vi "_test LoadUnload.vi"() -> ()   [LabVIEW 2020]
uses:
  C:/Users/Administrator/Desktop/GIT/Ballard-Arinc-429-XML-Generator/Source/Assemblies/Ballard_Parameter_ni/bin/Debug/Parameters_Arinc429_XML_Tools.dll
  Source/Assemblies/Ballard_Parameter_ni/bin/Debug/Parameters_Arinc429_XML_Tools.dll
panel:
  out "parameters":T1(array[cluster])
  out "error out":errorcluster
  in  "XML path":path=path "C:/Users/Administrator/Desktop/GIT/Ballard-Arinc-429-XML-Generator/Database Examples/Parameters.xml"
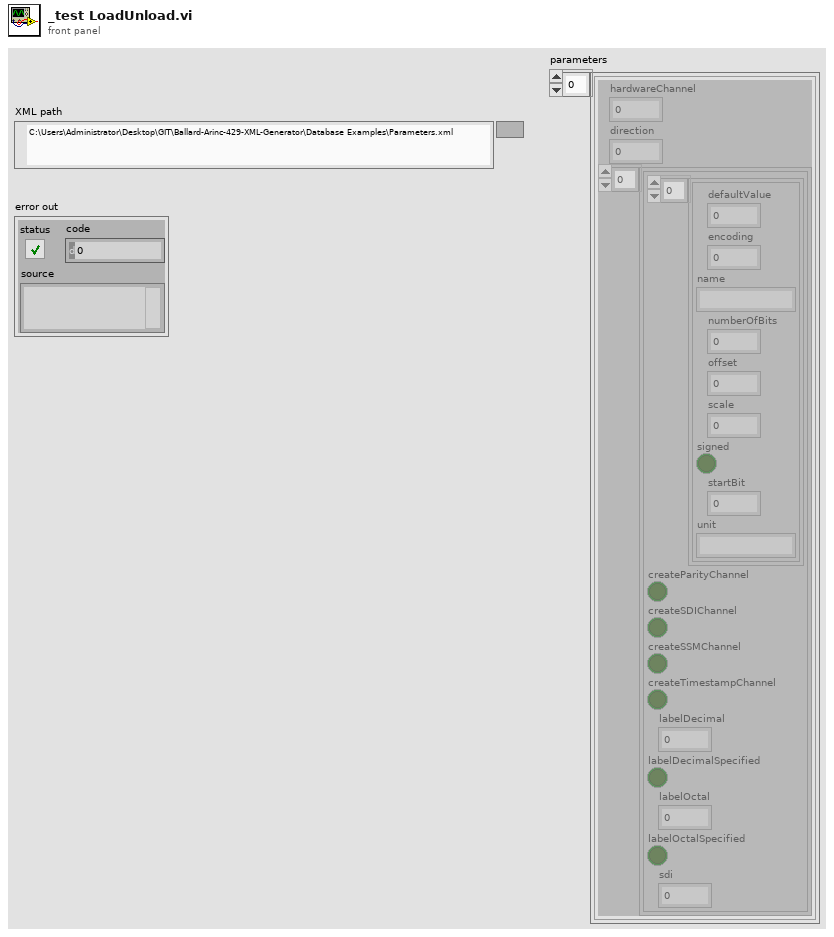
[diagram p1: front panel]
types:
  T1 = cluster{"hardwareChannel":i32, "direction":i32, cluster{cluster{"defaultValue":dbl, "encoding":i32, "name":string, "numberOfBits":i32, "offset":dbl, "scale":dbl, "signed":bool, "startBit":i32, "unit":string}[], "createParityChannel":bool, "createSDIChannel":bool, "createSSMChannel":bool, "createTimestampChannel":bool, "labelDecimal":i32, "labelDecimalSpecified":bool, "labelOctal":i32, "labelOctalSpecified":bool, "sdi":i32}[]}[]
  T2 = cluster{"defaultValue":dbl, "encoding":i32, "name":string, "numberOfBits":i32, "offset":dbl, "scale":dbl, "signed":bool, "startBit":i32, "unit":string}
  T3 = cluster{cluster{"defaultValue":dbl, "encoding":i32, "name":string, "numberOfBits":i32, "offset":dbl, "scale":dbl, "signed":bool, "startBit":i32, "unit":string}[], "createParityChannel":bool, "createSDIChannel":bool, "createSSMChannel":bool, "createTimestampChannel":bool, "labelDecimal":i32, "labelDecimalSpecified":bool, "labelOctal":i32, "labelOctalSpecified":bool, "sdi":i32}
  T4 = cluster{"hardwareChannel":i32, "direction":i32, cluster{cluster{"defaultValue":dbl, "encoding":i32, "name":string, "numberOfBits":i32, "offset":dbl, "scale":dbl, "signed":bool, "startBit":i32, "unit":string}[], "createParityChannel":bool, "createSDIChannel":bool, "createSSMChannel":bool, "createTimestampChannel":bool, "labelDecimal":i32, "labelDecimalSpecified":bool, "labelOctal":i32, "labelOctalSpecified":bool, "sdi":i32}[]}
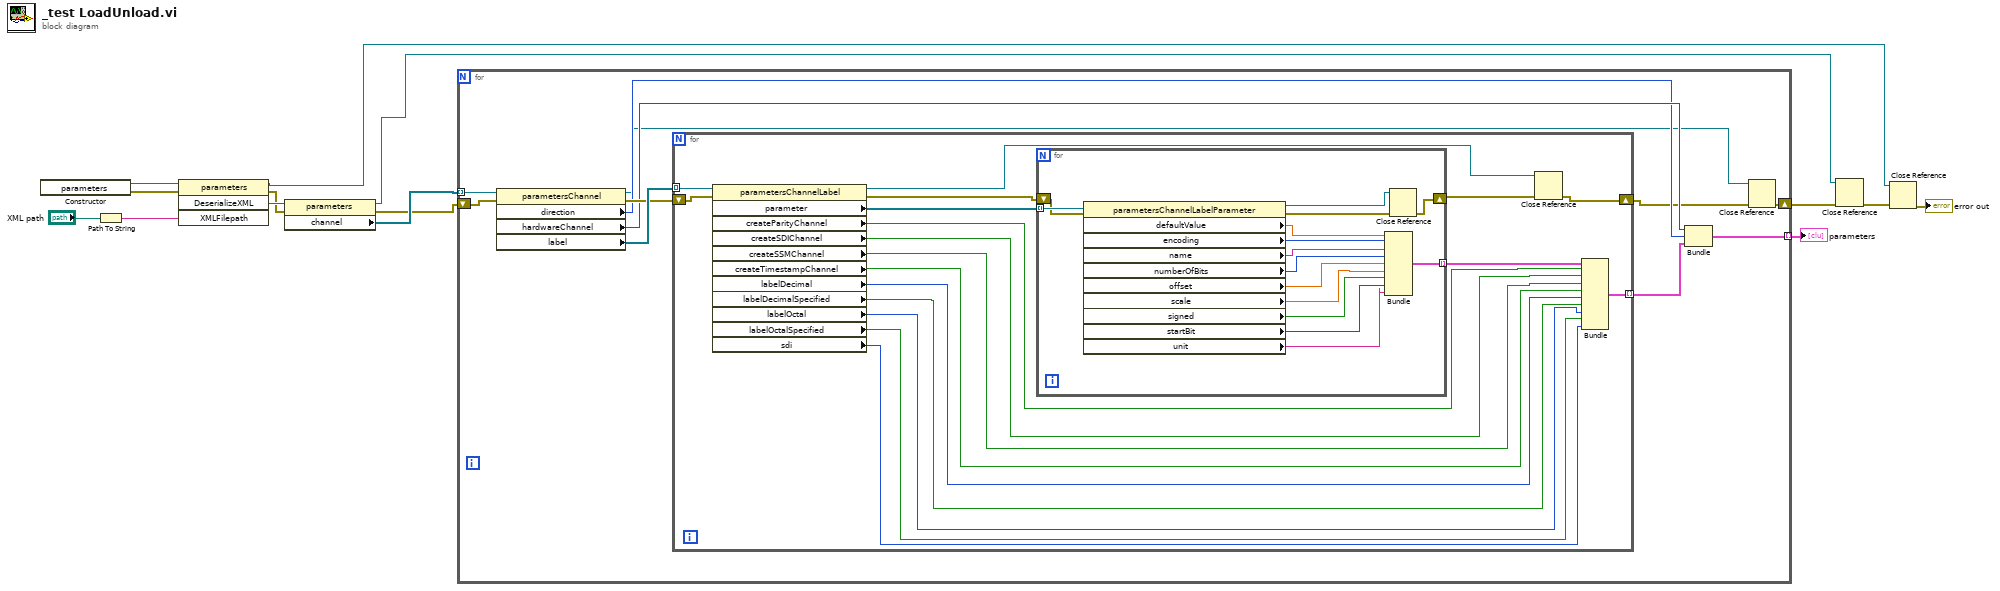
[diagram p0: block diagram]
diagram:
  n1 = constructor class="parameters"() -> (reference out=w14:refnum<k24>, error out=w13:errorcluster)  [unwired: 3 in, 1 out]
  n2 = Path To String(path="XML path") -> (string=w11:string)
  n3 = invoke class="parameters" method="DeserializeXML"(reference=w14, error in=w13, "XMLFilepath"=w11) -> (reference out=w3:refnum<k24>, error out=w9:errorcluster, "DeserializeXML"=w10:refnum<k24>)  [unwired: 1 in, 1 out]
  n4 = property class="parameters"(reference=w10, error in=w9) -> (reference out=w6:refnum<k24>, error out=w7:errorcluster, "channel"=w8:refnum<k24>[])
  n5 = for {
    tunnel: w8 -> [w25] mode=indexing
    shift-right: [w16] -> w5
    shift-left: w7 -> [w24]
    tunnel: [w15] -> w1 mode=indexing
    n6 = property class="parametersChannel"(reference=w25, error in=w24) -> (reference out=w18:refnum<k24>, error out=w22:errorcluster, "direction"=w20:i32, "hardwareChannel"=w21:i32, "label"=w23:refnum<k24>[])
    n7 = for {
      tunnel: w23 -> [w43] mode=indexing
      shift-right: [w26] -> w17
      shift-left: w22 -> [w42]
      tunnel: [w27] -> w19 mode=indexing
      n8 = property class="parametersChannelLabel"(reference=w43, error in=w42) -> (reference out=w39:refnum<k24>, error out=w41:errorcluster, "parameter"=w40:refnum<k24>[], "createParityChannel"=w36:bool, "createSDIChannel"=w35:bool, "createSSMChannel"=w34:bool, "createTimestampChannel"=w33:bool, "labelDecimal"=w32:i32, "labelDecimalSpecified"=w31:bool, "labelOctal"=w30:i32, "labelOctalSpecified"=w29:bool, "sdi"=w28:i32)
      n9 = for {
        tunnel: w40 -> [w58] mode=indexing
        tunnel: [w47] -> w37 mode=indexing
        shift-right: [w45] -> w38
        shift-left: w41 -> [w57]
        n10 = property class="parametersChannelLabelParameter"(reference=w58, error in=w57) -> (reference out=w44:refnum<k24>, error out=w46:errorcluster, "defaultValue"=w56:dbl, "encoding"=w55:i32, "name"=w54:string, "numberOfBits"=w53:i32, "offset"=w52:dbl, "scale"=w51:dbl, "signed"=w50:bool, "startBit"=w49:i32, "unit"=w48:string)
        n11 = Bundle("defaultValue"=w56, "encoding"=w55, "name"=w54, "numberOfBits"=w53, "offset"=w52, "scale"=w51, "signed"=w50, "startBit"=w49, "unit"=w48) -> (w47:T2)  [unwired: 1 in]
        n12 = Close Reference(reference=w44, error in (no error)=w46) -> (error out=w45:errorcluster)
      }
      n13 = Close Reference(reference=w39, error in (no error)=w38) -> (error out=w26:errorcluster)
      n14 = Bundle(w37, "createParityChannel"=w36, "createSDIChannel"=w35, "createSSMChannel"=w34, "createTimestampChannel"=w33, "labelDecimal"=w32, "labelDecimalSpecified"=w31, "labelOctal"=w30, "labelOctalSpecified"=w29, "sdi"=w28) -> (w27:T3)  [unwired: 1 in]
    }
    n15 = Bundle("hardwareChannel"=w21, "direction"=w20, w19) -> (w15:T4)  [unwired: 1 in]
    n16 = Close Reference(reference=w18, error in (no error)=w17) -> (error out=w16:errorcluster)
  }
  "parameters" <- w1
  n17 = Close Reference(reference=w6, error in (no error)=w5) -> (error out=w4:errorcluster)
  n18 = Close Reference(reference=w3, error in (no error)=w4) -> (error out=→"error out":errorcluster)
